vi "跳一跳屏幕控制.vi"() -> ()   [LabVIEW 2014]
uses:
  user32.dll
  <vilib>/vision/NI_Vision_Development_Module.lvlib
  <vilib>/Utility/inputDevices.llb/joystickAcquire.vi
panel:
  in  "偏置":sgl=3.0
  out "时间":sgl
  in  "系数":sgl=4.28
  out "Image":T1(plugin-control)
  out "lPrect":cluster{i32, i32, i32, i32}
  out "返回类型 3":i32 format="%x"
  out "错误输出 2":errorcluster caption="错误输出"
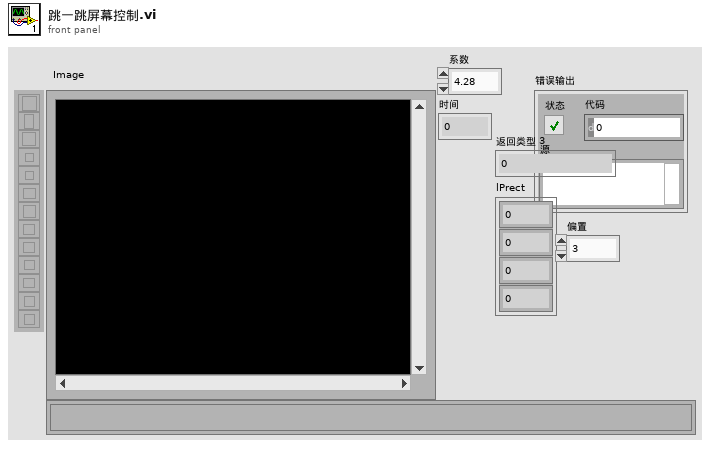
[diagram p1: front panel]
types:
  T1 = typedef "IMAQ Image.ctl" = refnum<image>
  T2 = typedef "Image Type" = u32
  T3 = cluster{"X axis":i32, "Y axis":i32, "Z axis":i32, "X axis rotation":i32, "Y axis rotation":i32, "Z axis rotation":i32, "U axis":i32, "V axis":i32}
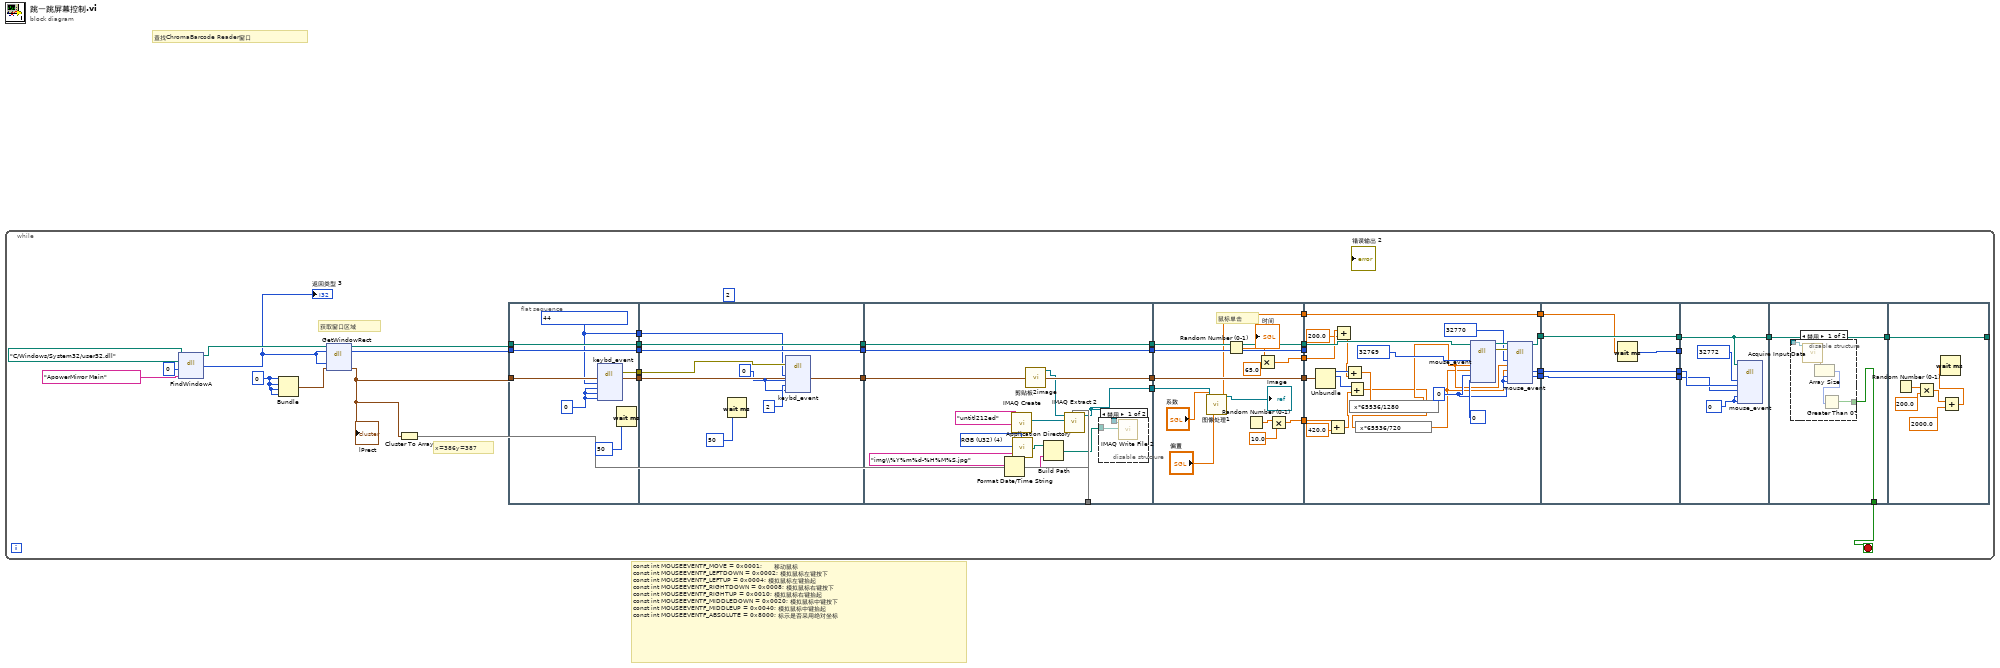
[diagram p0: block diagram]
diagram:
  # "const int MOUSEEVENTF_MOVE = 0x0001;      移动鼠标 \nconst int MOUSEEVENTF_LEFTDOWN = 0x0002; 模拟鼠标左键按下 \nconst int MOUSEEVENTF_LEFTUP = 0x0004; 模拟鼠标左键抬起 \nconst int MOUSEEVENTF_RIGHTDOWN = 0x0008; 模拟鼠标右键按下 \nconst int MOUSEEVENTF_RIGHTUP = 0x0010; 模拟鼠标右键抬起 \nconst int MOUSEEVENTF_MIDDLEDOWN = 0x0020; 模拟鼠标中键按下 \nconst int MOUSEEVENTF_MIDDLEUP = 0x0040; 模拟鼠标中键抬起 \nconst int MOUSEEVENTF_ABSOLUTE = 0x8000; 标示是否采用绝对坐标"
  # "查找ChromaBarcode Reader窗口"
  n1 = while {
    stop <- w3 stop-if-true
    (unwired) 2
    w13 = 0
    # "鼠标单击"
    # "x=386y=387"
    # "获取窗口区域"
    n2 = dll-call lib="C:/Windows/System32/user32.dll" fn="FindWindowA"(path in=path "C:/Windows/System32/user32.dll" ("路径输入"), "lpClassName"=0, "lpWindowName"="ApowerMirror Main") -> (path out=w14:path, "返回类型"=w10:i32)  [unwired: 4 in, 1 out]
    "返回类型 3" <- w10
    n3 = Bundle(w13, w13, w13, w13) -> (w12:cluster{i32, i32, i32, i32})  [unwired: 1 in]
    n4 = dll-call lib="C:/Windows/System32/user32.dll" fn="GetWindowRect"(path in=w14, "hwnd"=w10, "lPrect"=w12) -> (path out=w11:path, "lPrect"=w9:cluster{i32, i32, i32, i32})  [unwired: 4 in, 1 out]
    "lPrect" <- w9
    n5 = Cluster To Array(cluster=w9) -> (array=w8:i32[])
    n6 = flat-sequence {
      tunnel: w10 -> [w44]
      tunnel: w9 -> [w45]
      tunnel: w11 -> [w46]
      tunnel: [w46] -> w39
      tunnel: [w45] -> w38
      tunnel: [w44] -> w37
      tunnel: [w41] -> w36
      tunnel: [w40] -> w35
      tunnel: w39 -> [w54]
      tunnel: [w54] -> w34
      tunnel: w38 -> [w53]
      tunnel: [w53] -> w33
      tunnel: w37 -> [w52]
      tunnel: [w52] -> w32
      tunnel: w36 -> [w48]
      tunnel: w35 -> [w47]
      tunnel: w34 -> [w67]
      tunnel: [w67] -> w31
      tunnel: w33 -> [w66]
      tunnel: [w66] -> w30
      tunnel: w32 -> [w65]
      tunnel: [w65] -> w29
      tunnel: w8 -> [w61]
      tunnel: [w55] -> w28
      tunnel: w31 -> [w83]
      tunnel: [w83] -> w27
      tunnel: w30 -> [w82]
      tunnel: [w82] -> w26
      tunnel: w29 -> [w81]
      tunnel: [w81] -> w25
      tunnel: w28 -> [w74]
      tunnel: [w77] -> w5
      tunnel: [w75] -> w4
      tunnel: [w73] -> w1
      tunnel: [w99] -> w24
      tunnel: [w96] -> w23
      tunnel: [w95] -> w22
      tunnel: w27 -> [w101]
      tunnel: w26 -> [w107]
      tunnel: w25 -> [_]
      tunnel: w5 -> [w90]
      tunnel: w4 -> [w86]
      tunnel: [w84] -> w2
      tunnel: w1 -> [w84]
      tunnel: w24 -> [w111]
      tunnel: w23 -> [w110]
      tunnel: w22 -> [w109]
      tunnel: [w112] -> w21
      tunnel: [w111] -> w20
      tunnel: [w110] -> w19
      tunnel: [w109] -> w18
      tunnel: w2 -> [w108]
      tunnel: w21 -> [_]
      tunnel: w20 -> [w113]
      tunnel: w19 -> [w115]
      tunnel: w18 -> [w114]
      tunnel: [w113] -> w7
      tunnel: w7 -> [w119]
      tunnel: [w119] -> w6
      tunnel: [w118] -> w3
      tunnel: w6 -> [w129]
      tunnel: [w129] -> _
      frame #0 {
        w43 = u8 0 ("bScan")
        w40 = u16 44 ("Extended Virtual Key List")
        n7 = dll-call lib="user32.dll" fn="keybd_event"("bVk"=w40, "bScan"=w43, "dwFlags"=w43, "dwExtraInfo"=w43) -> (error out=w41:errorcluster)  [unwired: 4 in, 5 out]
        n8 = Wait (ms)(milliseconds to wait=u32 50 ("等待时间（毫秒）")) -> ()  [unwired: 1 out]
      }
      frame #1 {
        w50 = u8 0 ("bScan")
        n9 = Wait (ms)(milliseconds to wait=u32 50 ("等待时间（毫秒）")) -> ()  [unwired: 1 out]
        n10 = dll-call lib="user32.dll" fn="keybd_event"(error in=w48, "bVk"=w47, "bScan"=w50, "dwFlags"=u32 2, "dwExtraInfo"=w50) -> ()  [unwired: 4 in, 5 out]
      }
      frame #2 {
        w60 = T2 4 items=["Grayscale (U8)", "Grayscale (I16)", "Grayscale (SGL)", "Complex (CSG)", "RGB (U32)", "HSL (U32)", "RGB (U64)", "Grayscale (U16)"] ("Image Type")
        n11 = Format Date/Time String(time format string (%c)="img\\%Y%m%d-%H%M%S.jpg" ("时间格式字符串(%c)")) -> (date/time string=w57:string)  [unwired: 2 in]
        n12 = call "IMAQ Create"("Image Name"="untitl212ed", "Image Type"=w60) -> ("New Image"=w62:T1)  [unwired: 3 in, 1 out]
        n13 = call <vilib>:"Application Directory.vi"() -> ("Application Directory"=w58:path)
        n14 = call "剪贴板2image.vi"() -> ("Image Out 2"=w64:T1)  [unwired: 9 in, 2 out]
        n15 = Build Path(base path=w58, name or relative path=w57) -> (appended path=w56:path)
        n16 = call "IMAQ Extract 2"("Optional Rectangle"=w61, "Image Dst"=w62, "Image Src"=w64) -> ("Image Dst Out"=w55:T1)  [unwired: 7 in, 1 out]
        n17 = disable-structure shown="禁用" {
          disable-tunnel: w56 -> [w69 _]
          disable-tunnel: w55 -> [w68 _]
          frame Disabled {
            n18 = call-poly "IMAQ Write File 2"("File Path"=w69, "Image"=w68) -> ()  [unwired: 8 in, 2 out]
          }
          frame Enabled {
          }
        }
      }
      frame #3 {
        n19 = call "图像处理1.vi"("Image In"=w74, "系数"="系数", "偏置"="偏置") -> ("时间"=w73:sgl, "Image Out"=→"Image":T1)  [unwired: 23 in]
        n20 = Random Number (0-1)() -> (number: 0 to 1=w79:dbl)
        n21 = Random Number (0-1)() -> (number: 0 to 1=w76:dbl)
        n22 = Multiply(x=w79, y=65.0) -> (x*y=w77:dbl)
        n23 = Multiply(x=w76, y=10.0) -> (x*y=w75:dbl)
      }
      frame #4 {
        w97 = 0 ("dx")
        n24 = Unbundle(w107) -> (w106:i32, w105:i32)  [unwired: 2 out]
        n25 = Add(x=w86, y=420.0) -> (x+y=w85:dbl)
        n26 = Add(x=w90, y=200.0) -> (x+y=w88:dbl)
        n27 = Add(x=w106, y=w88) -> (x+y=w94:dbl)
        n28 = Add(x=w105, y=w85) -> (x+y=w92:dbl)
        n29 = expression code="x*65536/1280"(w94) -> (w93:dbl)
        n30 = expression code="x*65536/720"(w92) -> (w91:dbl)
        n31 = dll-call lib="user32.dll" fn="mouse_event"(path in=w101, "dwFlags"=32769, "dx"=w93, "dy"=w91, "cButtons"=w97, "dwExtraInfo"=0) -> (path out=w100:path, error out=w102:errorcluster)  [unwired: 8 in]
        n32 = dll-call lib="user32.dll" fn="mouse_event"(path in=w100, error in=w102, "dwFlags"=32770, "dx"=w93, "dy"=w91, "cButtons"=w97, "dwExtraInfo"=w97) -> (path out=w99:path, "dy"=w96:i32, "cButtons"=w95:i32)  [unwired: 5 in, 1 out]
      }
      frame #5 {
        n33 = Wait (ms)(milliseconds to wait=w108) -> (millisecond timer value=w112:u32)
      }
      frame #6 {
        w116 = 0 ("dwExtraInfo")
        n34 = dll-call lib="user32.dll" fn="mouse_event"(path in=w113, "dwFlags"=32772, "dx"=w115, "dy"=w114, "cButtons"=w116, "dwExtraInfo"=w116) -> ()  [unwired: 8 in, 2 out]
      }
      frame #7 {
        n35 = disable-structure shown="禁用" {
          disable-tunnel: _ -> [w123 _]
          disable-tunnel: [w120 _] -> w118
          frame Disabled {
            n36 = call-poly <vilib>:"Acquire Input Data.vi"("device ID"=w123) -> ("axis info"=w122:T3)  [unwired: 14 in, 4 out]
            n37 = Array Size(array=w122) -> (size(s)=w121:i32)
            n38 = Greater Than 0?(x=w121) -> (x > 0?=w120:bool)
          }
          frame Enabled {
          }
        }
      }
      frame #8 {
        n39 = Random Number (0-1)() -> (number: 0 to 1=w128:dbl)
        n40 = Multiply(x=w128, y=200.0) -> (x*y=w126:dbl)
        n41 = Add(x=w126, y=2000.0) -> (x+y=w124:dbl)
        n42 = Wait (ms)(milliseconds to wait=w124) -> ()  [unwired: 1 out]
      }
    }
  }
